vi "Main.vi"(11 "Module Admin":refnum<class "Delacor_lib_QMH_Module Admin.lvclass">) -> ()   [LabVIEW 2024, in "GUI.lvlib"]
doc: "This template is based off of the Queued Message Handler design pattern and the Queued Message Handler project template that ships with LabVIEW.\n\nThe main difference is that the queue is private to this module and communication between modules is performed via Broadcast and Request events.\n\nRequest events are wrapped in public API methods and are handled in the Event Handling Loop (EHL) of this VI. Any module can register for Broadcast events sent by this module. The EHL generates messages based on user interface actions.\n\nThe Message Handling Loop (MHL) processes messages generated by the EHL, or by other messages. The messages are string values, so new messages can be added easily to the Message Cases case structure in the MHL. Each message cluster can also provide an optional value for Message Data, which is a variant that can be converted to whatever message-specific data is required.\n_____\nBased on DQMH Dev Tools: Project Template 7.1.0.1503."
uses:
  GUI.lvlib
  <vilib>/Delacor/Delacor QMH/Libraries/Module Admin_class/Delacor_lib_QMH_Module Admin.lvclass
  DB/Controls/Login info.ctl
  DB/Controls/User level.ctl
  Controls/Main Buttons.ctl
  Controls/Settings.ctl
  <vilib>/vision/Instrument.llb/QR Code Description Options.ctl
  <vilib>/vision/Instrument.llb/Data Matrix Polarity.ctl
  <vilib>/vision/Instrument.llb/QR Code Model Type.ctl
  Controls/HW Status.ctl
  Module Data--cluster.ctl
  <vilib>/Delacor/Delacor QMH/Libraries/Message Queue_class/Delacor_lib_QMH_Message Queue.lvclass/Delacor_lib_QMH_Message Queue.ctl
  Stop Argument--cluster.ctl
  <vilib>/Delacor/Delacor QMH/Libraries/Module Admin_class/Delacor_lib_QMH_Module Admin.lvclass/Delacor_lib_QMH_Module Admin.ctl
  login Argument--cluster.ctl
  login_ Argument--cluster.ctl
  logout Argument--cluster.ctl
  Load settings Argument--cluster.ctl
  update serials array Argument--cluster.ctl
  update parent Argument--cluster.ctl
  update HW status indicator Argument--cluster.ctl
  Controls/HW Modules.ctl
  <vilib>/Utility/miscctls.llb/LVPointTypeDef.ctl
  GUI data ref.ctl
  <vilib>/Delacor/Delacor QMH/Libraries/Message Queue_class/Delacor_lib_QMH_Enqueue Message (Single).vi
  <vilib>/Delacor/Delacor QMH/Libraries/Module Admin_class/Delacor_lib_QMH_Get External Launch.vi
  <vilib>/Delacor/Delacor QMH/Libraries/Message Queue_class/Delacor_lib_QMH_Message Queue.lvclass
  DB/DB.lvlib
  Controller/Controller.lvlib
  PLC/PLC.lvlib
  Handheld Scanner/Handheld Scanner.lvlib
  Aggregation 1/Aggregation 1.lvlib
panel:
  in  "Close":bool
  in  "Back":bool
  out "Login info":T1
  in  "Tab Control":T3(tab)
  in  "Main buttons":T4
  out "Parent 2":string
  out "Parent 1":string
  in  "Start Tool":bool
  in  "Start Tool":bool
  out "Level 2 Serials":string[](array[string])
  out "Level 1 Serials":string[](array[string])
  out "Camera 2":T5(plugin-control)
  out "Camera 1":T5(plugin-control)
  out "Status":T6
  in  "Settings":T7
  in  "Cancel settings":bool
  in  "Save settings":bool
  out "Image":T5(plugin-control)
  in  "QR Search options":T8
  in  "QR Description Options":T9={"Matrix Size (cells)"=0, "Barcode Polarity"=-2, "Mirror Mode"=-2, "QR Model"=0} {"Mirror Mode" items=["Auto-detect"=-2, "Normal"=0, "Mirrored"=1]; "Matrix Size (cells)" items=["Auto-detect"=0, "11x11 - Version 1 (Micro QR Only)"=11, "13x13 - Version 2 (Micro QR Only)"=13, "15x15 - Version 3 (Micro QR Only)"=15, "17x17 - Version 4 (Micro QR Only)"=17, "21x21 - Version 1"=21, "25x25 - Version 2"=25, "29x29 - Version 3"=29, "33x33 - Version 4"=33, "37x37 - Version 5"=37, "41x41 - Version 6"=41, "45x45 - Version 7"=45, "49x49 - Version 8"=49, "53x53 - Version 9"=53, "57x57 - Version 10"=57, "61x61 - Version 11"=61, "65x65 - Version 12"=65, "69x69 - Version 13"=69, "73x73 - Version 14"=73, "77x77 - Version 15"=77, "81x81 - Version 16"=81, "85x85 - Version 17"=85, "89x89 - Version 18"=89, "93x93 - Version 19"=93, "97x97 - Version 20"=97, "101x101 - Version 21"=101, "105x105 - Version 22"=105, "109x109 - Version 23"=109, "113x113 - Version 24"=113, "117x117 - Version 25"=117, "121x121 - Version 26"=121, "125x125 - Version 27"=125, "129x129 - Version 28"=129, "133x133 - Version 29"=133, "137x137 - Version 30"=137, "141x141 - Version 31"=141, "145x145 - Version 32"=145, "149x149 - Version 33"=149, "153x153 - Version 34"=153, "157x157 - Version 35"=157, "161x161 - Version 36"=161, "165x165 - Version 37"=165, "169x169 -  Version 38"=169, "173x173 - Version 39"=173, "177x177 - Version 40"=177]; "QR Model" items=["Auto-detect", "Micro", "Model 1", "Model 2"]; "Barcode Polarity" items=["Auto-detect"=-2, "Black on White"=0, "White on Black"=1]}
  out "error out":errorcluster
  out "Status":string
  in  "Simulate MHL Error":bool
  in  "Simulate EHL Error":bool
  # "Other processes communicate with this Module via its Public API (wrappers for its Request Events).\n\nThis Module communicates with other processes via its Broadcast Events.\nAny process that wants to receive these messages can register for this module's Broadcast events."
  # "This template is for the DQMH framework. See the block diagram for more information on how to use this template."
  # "No User logged in\n        Or Database Not Connected\n\nPlease Login from Serialization System"
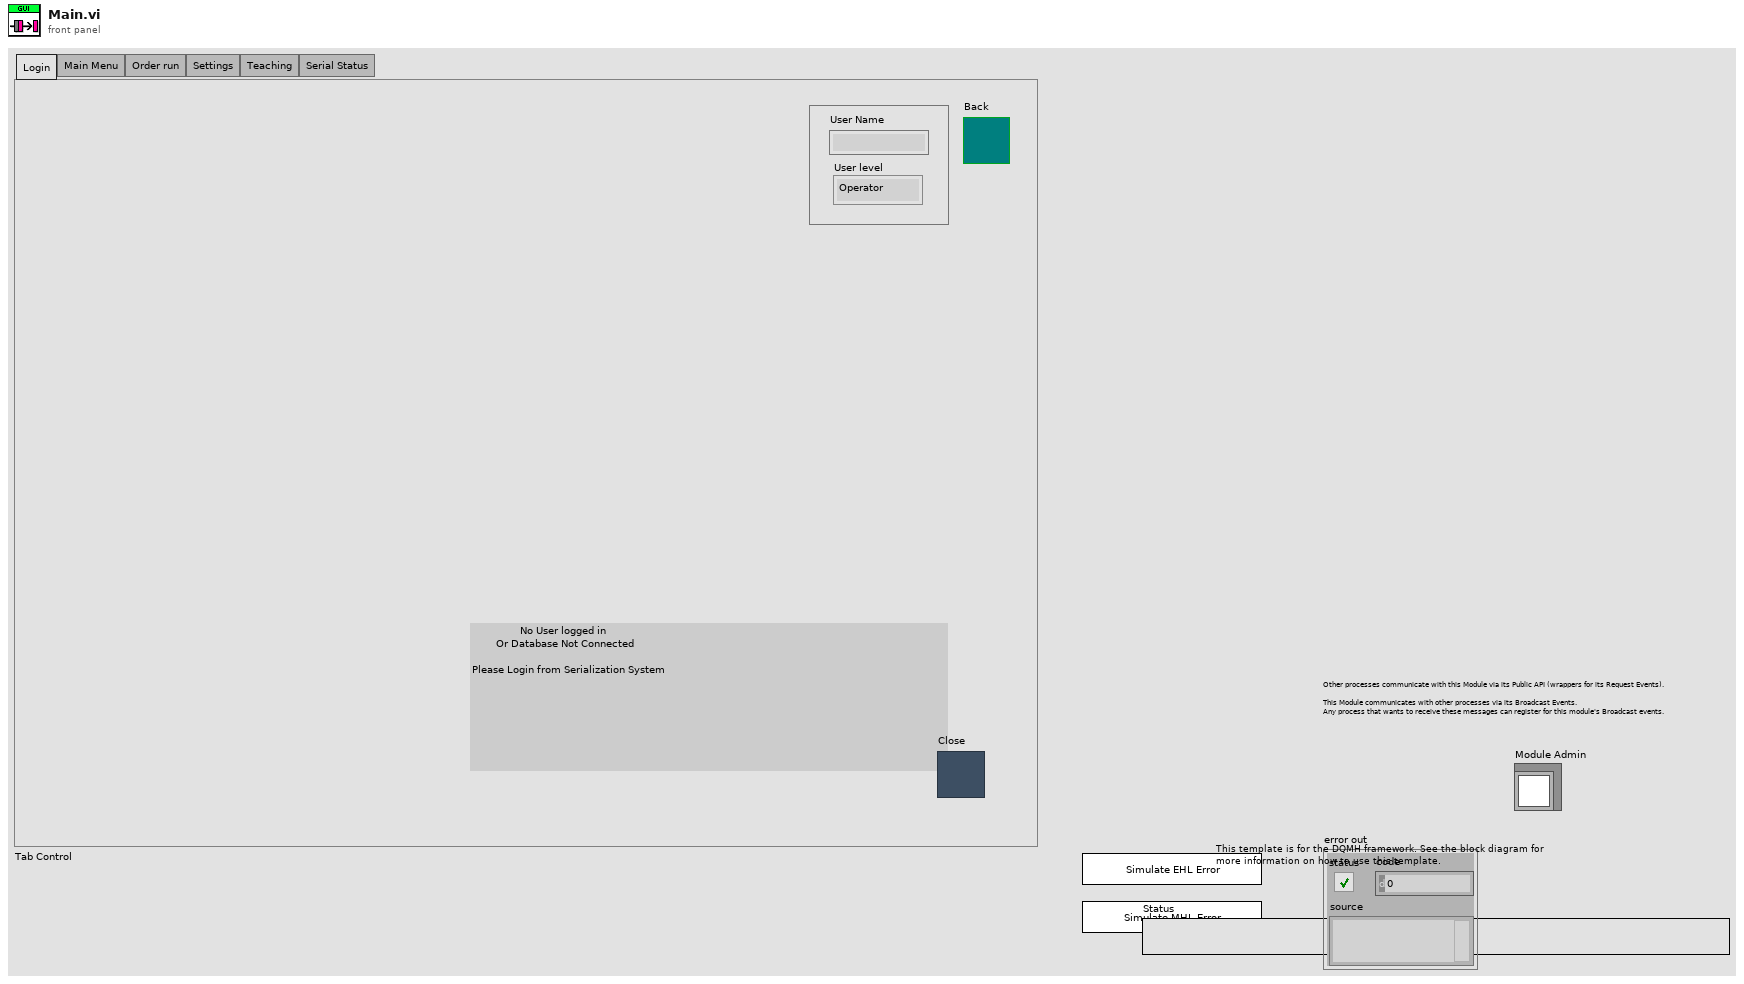
[diagram p1: front panel]
types:
  T1 = typedef "Login info.ctl" = cluster{"User Name":string, "User level":T2}
  T2 = typedef "User level.ctl" = enum16{"Operator", "Admin"}
  T3 = enum32{"Login", "Main Menu", "Order run", "Settings", "Teaching", "Serial Status"}
  T4 = typedef "Main Buttons.ctl" = cluster{"Start Button":bool, "Tools Button":bool, "Teaching Button":bool, "Serial Status Button":bool}
  T5 = typedef "IMAQ Image.ctl" = refnum<image>
  T6 = typedef "HW Status.ctl" = cluster{"Cam 1":bool, "Cam 2":bool, "Printer 1":bool, "Printer 2":bool, "PLC":bool, "Level 2 scanner":bool, "Handheld scanner":bool}
  T7 = typedef "Settings.ctl" = cluster{"Camera 1 IP":string, "Camera 2 IP":string, "Printer 1 IP":string, "Printer 2 IP":string, "Level 2 Scanner COM":refnum<visa-resource-name>, "PLC Port":dbl, "PLC IP":string, "Handheld Scanner COM":refnum<visa-resource-name>, "Printer2 Port":dbl, "Cam1 send port ":dbl, "Cam1 recv port":dbl, "Cam2 send port":dbl, "Cam recv port":dbl, "Printer1 Port":dbl}
  T8 = cluster{"Rotation Mode":enum32{"Unlimited", "0 Degrees", "90 Degrees", "180 Degrees", "270 Degrees"}, "Skip Location?":bool, "Edge Threshold":u32, "Demodulation Mode":i32, "Cell Sample Size":i32, "Cell Filter Mode":i32, "Skew Degrees Allowed":u32}
  T9 = typedef "QR Code Description Options.ctl" = cluster{"Matrix Size (cells)":i32, "Barcode Polarity":T10, "Mirror Mode":i32, "QR Model":T11}
  T10 = typedef "Data Matrix Polarity.ctl" = i32
  T11 = typedef "QR Code Model Type.ctl" = i32
  T12 = typedef "Controller.lvlib/Broadcast Events--cluster.ctl" = cluster{"Module Did Init":refnum<user-event>, "Status Updated":refnum<user-event>, "Error Reported":refnum<user-event>, "Module Did Stop":refnum<user-event>, "Update Module Execution Status":refnum<user-event>}
  T13 = typedef "DB.lvlib/Broadcast Events--cluster.ctl" = cluster{"Module Did Init":refnum<user-event>, "Status Updated":refnum<user-event>, "Error Reported":refnum<user-event>, "Module Did Stop":refnum<user-event>, "Update Module Execution Status":refnum<user-event>}
  T14 = typedef "PLC.lvlib/Broadcast Events--cluster.ctl" = cluster{"Module Did Init":refnum<user-event>, "Status Updated":refnum<user-event>, "Error Reported":refnum<user-event>, "Module Did Stop":refnum<user-event>, "Update Module Execution Status":refnum<user-event>}
  T15 = typedef "Aggregation 1.lvlib/Broadcast Events--cluster.ctl" = cluster{"Module Did Init":refnum<user-event>, "Status Updated":refnum<user-event>, "Error Reported":refnum<user-event>, "Module Did Stop":refnum<user-event>, "Update Module Execution Status":refnum<user-event>}
  T16 = typedef "Handheld Scanner.lvlib/Broadcast Events--cluster.ctl" = cluster{"Module Did Init":refnum<user-event>, "Status Updated":refnum<user-event>, "Error Reported":refnum<user-event>, "Module Did Stop":refnum<user-event>, "Update Module Execution Status":refnum<user-event>}
  T17 = typedef "GUI.lvlib/Request Events--cluster.ctl" = cluster{"Stop Module":refnum<user-event>, "Show Panel":refnum<user-event>, "Hide Panel":refnum<user-event>, "Get Module Execution Status":refnum<user-event>, "Show Diagram":refnum<user-event>, "login":refnum<user-event>, "login_":refnum<user-event>, "logout":refnum<user-event>, "Load settings":refnum<user-event>, "update serials array":refnum<user-event>, "update parent":refnum<user-event>, "update HW status indicator":refnum<user-event>}
  T18 = typedef "GUI.lvlib/Module Data--cluster.ctl" = cluster{"Status":string}
  T19 = enum32{"invalid lock state", "Not Locked", "Locked (No Password)", "Password-protected"}
  T20 = typedef "GUI.lvlib/Stop Argument--cluster.ctl" = cluster{"Origin":string, "Exit via Stop Module Req?":bool, "Wait for Module to stop?":bool}
  T21 = enum32{"Login", "Main Menu", "Order run", "Settings"}
  T22 = typedef "GUI.lvlib/login Argument--cluster.ctl" = cluster{"Login info":T1}
  T23 = typedef "GUI.lvlib/login_ Argument--cluster.ctl" = cluster{"Login info":T1}
  T24 = typedef "GUI.lvlib/logout Argument--cluster.ctl" = cluster{"Boolean":bool}
  T25 = typedef "GUI.lvlib/Load settings Argument--cluster.ctl" = cluster{"Settings":T7, "reconnect":bool}
  T26 = typedef "GUI.lvlib/update serials array Argument--cluster.ctl" = cluster{"serial array":string[], "level":dbl}
  T27 = typedef "GUI.lvlib/update parent Argument--cluster.ctl" = cluster{"Parent":string, "level":dbl}
  T28 = typedef "GUI.lvlib/update HW status indicator Argument--cluster.ctl" = cluster{"HW Module":T29, "Status":bool}
  T29 = typedef "HW Modules.ctl" = string
  T30 = typedef "LVPointTypeDef.ctl" = cluster{"Horizontal":i16, "Vertical":i16}
  T31 = enum32{"Invalid", "Standard", "Closed", "Hidden", "Minimized", "Maximized"}
  T32 = typedef "GUI data ref.ctl" = cluster{"Printer 1 IP":refnum<vi>, "Camera 2 IP":refnum<vi>, "Camera 1 IP":refnum<vi>, "Printer 2 IP":refnum<vi>}
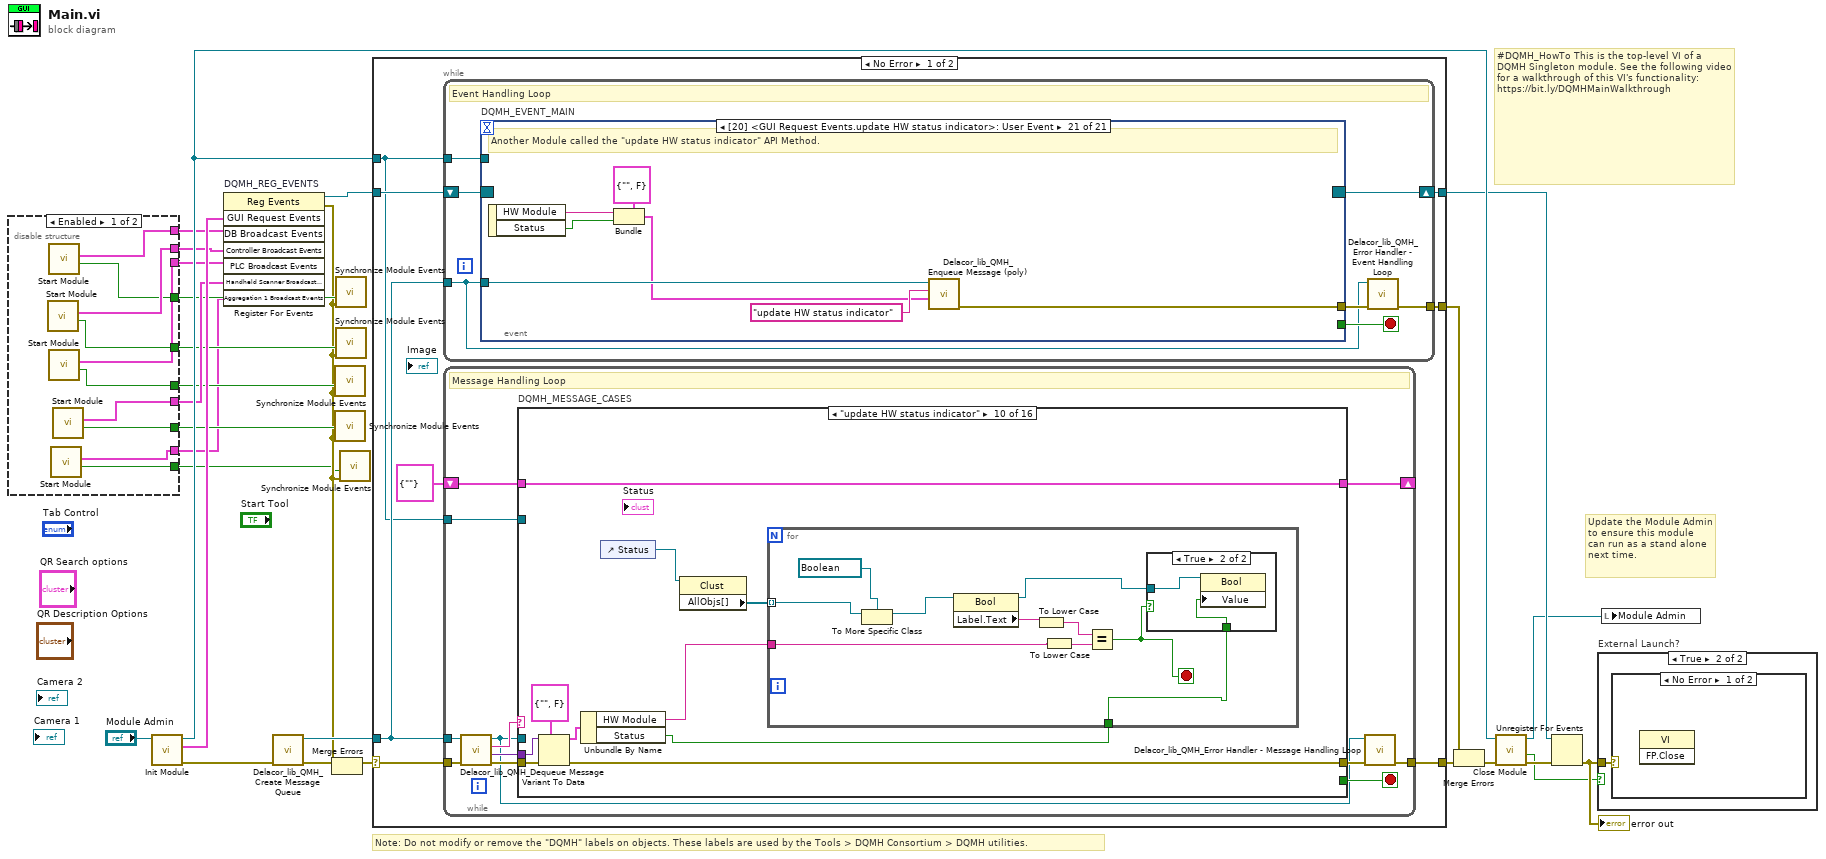
[diagram p0: block diagram]
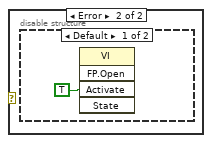
[diagram p4: hidden frame]
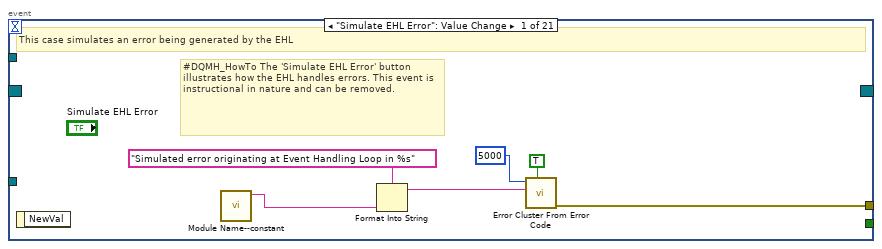
[diagram p6: hidden frame]
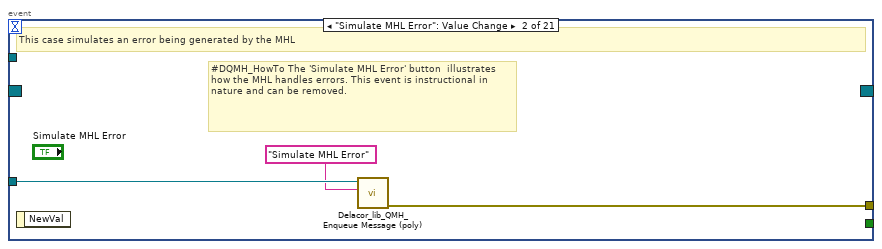
[diagram p7: hidden frame]
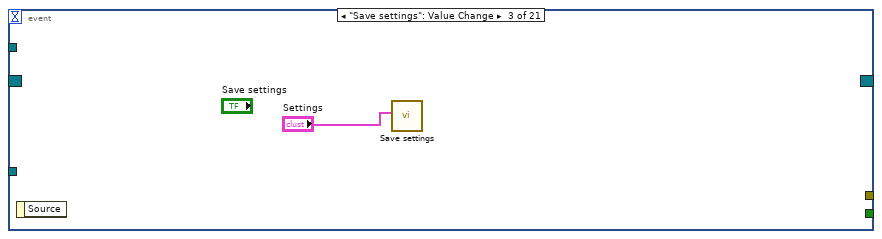
[diagram p8: hidden frame]
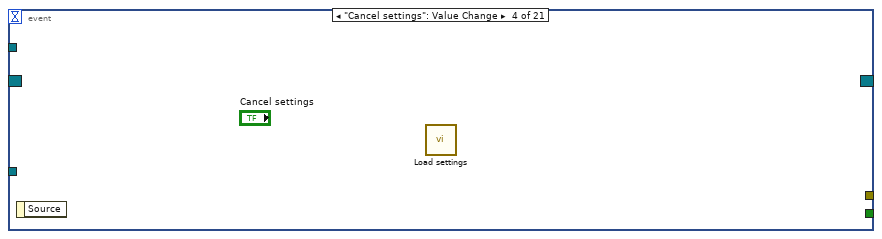
[diagram p9: hidden frame]
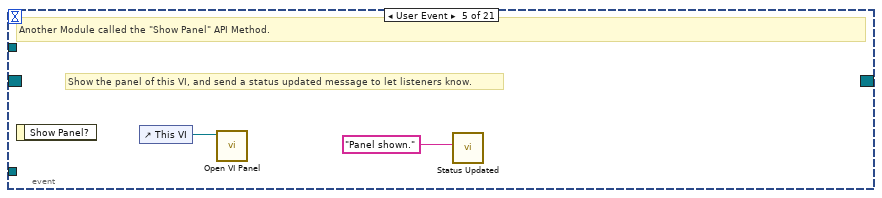
[diagram p10: hidden frame]
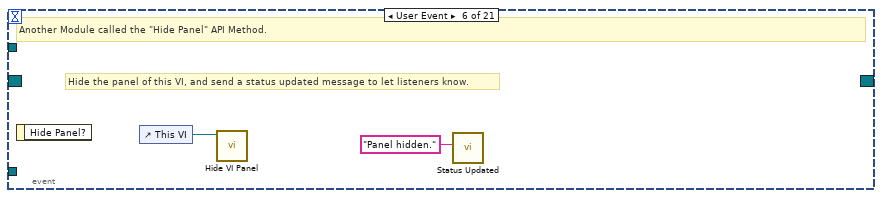
[diagram p11: hidden frame]
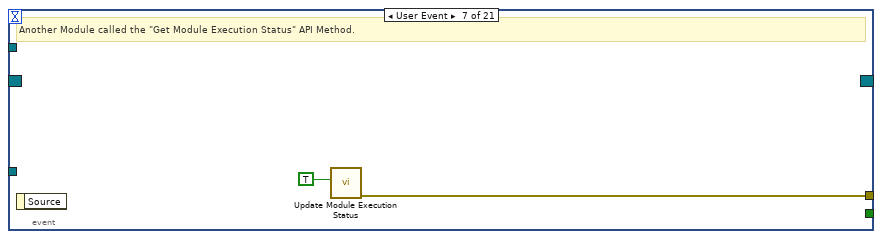
[diagram p12: hidden frame]
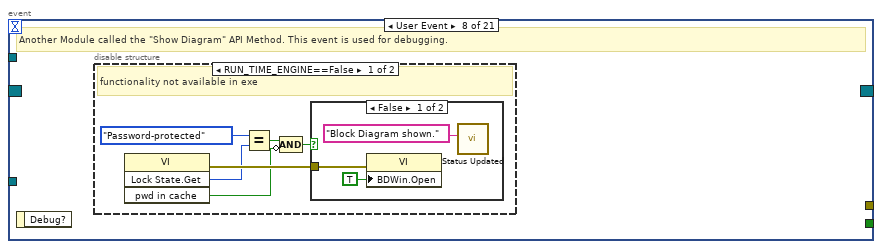
[diagram p13: hidden frame]
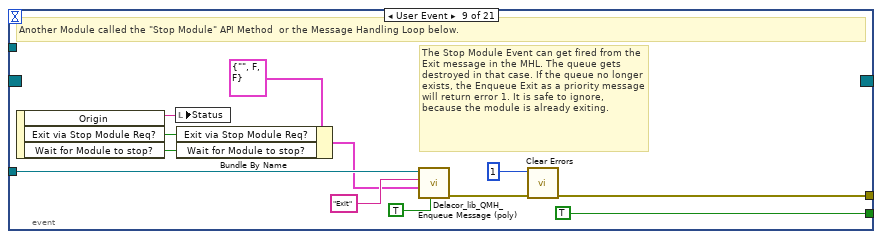
[diagram p16: hidden frame]
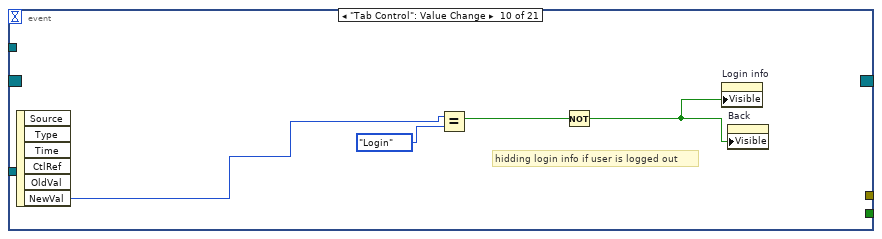
[diagram p17: hidden frame]
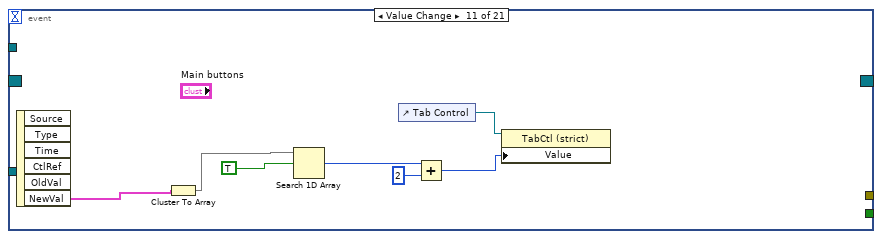
[diagram p18: hidden frame]
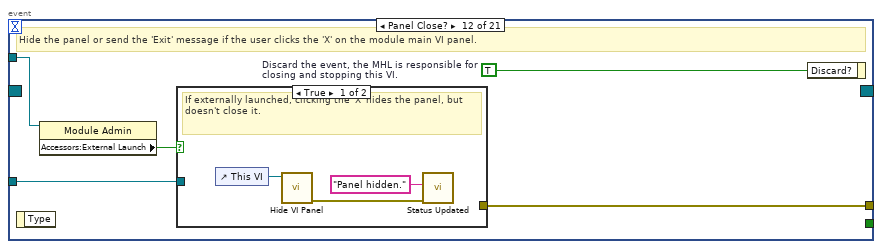
[diagram p19: hidden frame]
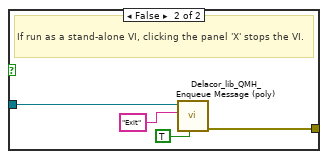
[diagram p20: hidden frame]
diagram:
  # "#DQMH_HowTo This is the top-level VI of a DQMH Singleton module. See the following video for a walkthrough of this VI's functionality: https://bit.ly/DQMHMainWalkthrough"
  # "Note: Do not modify or remove the \"DQMH\" labels on objects. These labels are used by the Tools > DQMH Consortium > DQMH utilities."
  # "Update the Module Admin to ensure this module can run as a stand alone next time."
  n1 = disable-structure shown="Enabled" {
    disable-tunnel: [w37 _] -> w11
    disable-tunnel: [w36 _] -> w10
    disable-tunnel: [w35 _] -> w9
    disable-tunnel: [w34 _] -> w8
    disable-tunnel: [w33 _] -> w7
    disable-tunnel: [w32 _] -> w6
    disable-tunnel: [w31 _] -> w5
    disable-tunnel: [w30 _] -> w4
    disable-tunnel: [w29 _] -> w2
    disable-tunnel: [w28 _] -> w1
    frame Enabled {
      n2 = call "Start Module.vi"() -> ("Wait for Event Sync?"=w32:bool, "Controller Broadcast Events"=w36:T12)  [unwired: 7 in, 3 out]
      n3 = call "Start Module.vi"() -> ("Wait for Event Sync?"=w33:bool, "DB Broadcast Events"=w37:T13)  [unwired: 7 in, 3 out]
      n4 = call "Start Module.vi"() -> ("Wait for Event Sync?"=w31:bool, "PLC Broadcast Events"=w35:T14)  [unwired: 7 in, 3 out]
      n5 = call "Start Module.vi"() -> ("Wait for Event Sync?"=w29:bool, "Aggregation 1 Broadcast Events"=w28:T15)  [unwired: 7 in, 3 out]
      n6 = call "Start Module.vi"() -> ("Wait for Event Sync?"=w30:bool, "Handheld Scanner Broadcast Events"=w34:T16)  [unwired: 7 in, 3 out]
    }
    frame Disabled {
    }
  }
  n7 = call "Init Module.vi"("Singleton Module Admin in"="Module Admin") -> ("error out"=w26:errorcluster, "GUI Request Events"=w16:T17, "Singleton Module Admin out"=w19:refnum<class "Delacor_lib_QMH_Module Admin.lvclass">)  [unwired: 8 in]
  n8 = register-events "DQMH_REG_EVENTS"(w16, w11, w10, w9, w8, w1) -> (reference out=w17:refnum<event-registration>, error out=w3:errorcluster)  [unwired: 2 in]
  n9 = call <vilib>:"Delacor_lib_QMH_Create Message Queue.vi"("error in"=w26) -> ("error out"=w21:errorcluster, "Message Queue"=w15:refnum<class "Delacor_lib_QMH_Message Queue.lvclass">)  [unwired: 9 in]
  n10 = Merge Errors(w21, w3) -> (w20:errorcluster)
  n11 = call "Synchronize Module Events.vi"("error in"=w3, "Wait for Event Sync?"=w5) -> ()  [unwired: 9 in, 1 out]
  n12 = call "Synchronize Module Events.vi"("error in"=w3, "Wait for Event Sync?"=w4) -> ()  [unwired: 9 in, 1 out]
  n13 = call "Synchronize Module Events.vi"("error in"=w3, "Wait for Event Sync?"=w7) -> ()  [unwired: 9 in, 1 out]
  n14 = call "Synchronize Module Events.vi"("error in"=w3, "Wait for Event Sync?"=w6) -> ()  [unwired: 9 in, 1 out]
  n15 = call "Synchronize Module Events.vi"("error in"=w3, "Wait for Event Sync?"=w2) -> ()  [unwired: 9 in, 1 out]
  n16 = case shown="No Error" w20 {
    selector: w20 -> [w43 w352]
    tunnel: [w45 w351] -> w27
    tunnel: [w42 w350] -> w18
    tunnel: w17 -> [w40 w350]
    tunnel: w15 -> [w39 w345]
    tunnel: [w44 _] -> w24
    tunnel: w19 -> [w38 w346]
    frame No Error {
      n17 = while {
        tunnel: w39 -> [w46]
        shift-right: [w49] -> w42
        shift-left: w40 -> [w50]
        tunnel: [w51] -> w44
        tunnel: w38 -> [w47]
        stop <- w48 stop-if-true
        # "Event Handling Loop"
        n18 = event "DQMH_EVENT_MAIN" shown="[20] <GUI Request Events.update HW status indicator>: User Event" {
          selector: w50 -> [_ _ _ _ _ _ _ _ _ _ _ _ _ _ _ _ _ _ _ _ _]
          dyn-events: [_ _ _ _ _ _ _ _ _ _ _ _ _ _ _ _ _ _ _ _ _] -> w49
          timeout: _ -> [_ _ _ _ _ _ _ _ _ _ _ _ _ _ _ _ _ _ _ _ _]
          tunnel: [_ _ _ _ _ _ _ _ TRUE ("Discard?") _ _ _ _ _ _ _ _ _ _ _ _] -> w48
          tunnel: w46 -> [_ w60 _ _ _ _ _ _ w85 _ _ w103 _ w118 w124 w130 _ w142 w149 w156 w163]
          tunnel: [w58 w61 _ _ _ _ w68 _ w88 _ _ w105 _ w113 w119 w125 _ w137 w143 w150 w157] -> w52
          tunnel: w47 -> [_ _ _ _ _ _ _ _ _ _ _ w102 _ _ _ _ _ _ _ _ _]
          event "Simulate EHL Error": Value Change {
            # "#DQMH_HowTo The 'Simulate EHL Error' button  illustrates how the EHL handles errors. This event is instructional in nature and can be removed."
            # "This case simulates an error being generated by the EHL"
            n19 = event-data() -> ()  [unwired: 1 in, 1 out]
            n20 = call "Module Name--constant.vi"() -> ("Module Name"=w55:string)  [unwired: 11 in]
            n21 = Format Into String(format string="Simulated error originating at Event Handling Loop in %s", w55) -> (resulting string=w56:string)  [unwired: 2 in, 1 out]
            n22 = call <vilib>:"Error Cluster From Error Code.vi"("show call chain? (False)"=TRUE, "error message (\"\")"=w56, "error code (0)"=5000) -> ("error out"=w58:errorcluster)  [unwired: 6 in]
          }
          event "Simulate MHL Error": Value Change {
            # "#DQMH_HowTo The 'Simulate MHL Error' button  illustrates how the MHL handles errors. This event is instructional in nature and can be removed."
            # "This case simulates an error being generated by the MHL"
            n23 = event-data() -> ()  [unwired: 1 in, 1 out]
            n24 = call-poly <vilib>:"Delacor_lib_QMH_Enqueue Message (poly).vi"("Message"="Simulate MHL Error", "Message Queue in"=w60) -> ("error out"=w61:errorcluster)  [unwired: 8 in, 1 out]
          }
          event "Save settings": Value Change {
            n25 = event-data() -> ()  [unwired: 1 in, 1 out]
            n26 = call "Save settings.vi"("Settings"="Settings") -> ()  [unwired: 10 in, 1 out]
          }
          event "Cancel settings": Value Change {
            n27 = event-data() -> ()  [unwired: 1 in, 1 out]
            n28 = call "Load settings.vi"() -> ()  [unwired: 11 in, 1 out]
          }
          event User Event {
            # "Show the panel of this VI, and send a status updated message to let listeners know."
            # "Another Module called the \"Show Panel\" API Method."
            n29 = event-data() -> ()  [unwired: 1 in, 1 out]
            n30 = control-ref of="This VI"() -> (w64:refnum<vi>)
            n31 = call "Open VI Panel.vi"("VI"=w64) -> ()  [unwired: 10 in, 1 out]
            n32 = call "Status Updated.vi"("Status"="Panel shown." ("format string")) -> ()  [unwired: 10 in, 1 out]
          }
          event User Event {
            # "Hide the panel of this VI, and send a status updated message to let listeners know."
            # "Another Module called the \"Hide Panel\" API Method."
            n33 = event-data() -> ()  [unwired: 1 in, 1 out]
            n34 = control-ref of="This VI"() -> (w66:refnum<vi>)
            n35 = call "Hide VI Panel.vi"("VI"=w66) -> ()  [unwired: 10 in, 1 out]
            n36 = call "Status Updated.vi"("Status"="Panel hidden." ("format string")) -> ()  [unwired: 10 in, 1 out]
          }
          event User Event {
            # "Another Module called the \"Get Module Execution Status\" API Method."
            n37 = event-data() -> ()  [unwired: 1 in, 1 out]
            n38 = call "Update Module Execution Status.vi"("Running?"=TRUE) -> ("error out"=w68:errorcluster)  [unwired: 10 in]
          }
          event User Event {
            # "Another Module called the \"Show Diagram\" API Method. This event is used for debugging."
            n39 = event-data() -> ()  [unwired: 1 in, 1 out]
            n40 = disable-structure shown="RUN_TIME_ENGINE==False" {
              frame condition #0 (active) {
                # "functionality not available in exe"
                n41 = invoke on="Invoke Node" class="VI" method="Lock State.Get"() -> (error out=w74:errorcluster, "Get Lock State"=w73:T19, "pwd in cache"=w70:bool)  [unwired: 4 in, 1 out]
                n42 = Equal?(x=T19."Password-protected", y=w73) -> (x = y?=w71:bool)
                n43 = Compound Arithmetic op=AND(w71, invert w70) -> (w69:bool)
                n44 = case shown="False" w69 {
                  tunnel: w74 -> [w77 _]
                  frame False {
                    n45 = property on="Property Node" class="VI"(error in=w77, "BDWin.Open"=TRUE ("Block Diagram Window:Open")) -> ()  [unwired: 1 in, 2 out]
                    n46 = call "Status Updated.vi"("Status"="Block Diagram shown." ("format string")) -> ()  [unwired: 10 in, 1 out]
                  }
                  frame True {
                    # "Password-protected VI, and the password is not in the cache. Do not show the diagram."
                  }
                }
              }
              frame condition #1 {
              }
            }
          }
          event User Event {
            # "The Stop Module Event can get fired from the Exit message in the MHL. The queue gets destroyed in that case. If the queue no longer exists, the Enqueue Exit as a priority message will return error 1. It is safe to ignore, because the module is already exiting."
            # "Another Module called the \"Stop Module\" API Method  or the Message Handling Loop below."
            n47 = event-data() -> ("Origin"=w84:string, "Exit via Stop Module Req?"=w80:bool, "Wait for Module to stop?"=w79:bool)  [unwired: 1 in]
            n48 = local write "Status"(w84) -> ()
            n49 = Bundle By Name(cluster=T20 {"Origin"="", "Exit via Stop Module Req?"=FALSE, "Wait for Module to stop?"=FALSE} ("Stop Argument"), "Exit via Stop Module Req?"=w80, "Wait for Module to stop?"=w79) -> (w78:T20)
            n50 = call-poly <vilib>:"Delacor_lib_QMH_Enqueue Message (poly).vi"("Priority Message? (F)"=TRUE, "Message Data"=w78, "Message"="Exit", "Message Queue in"=w85) -> ("error out"=w89:errorcluster)  [unwired: 6 in, 1 out]
            n51 = call <vilib>:"Clear Errors.vi"("error in (no error)"=w89, "specific error code to clear (0: all)"=1) -> ("error out"=w88:errorcluster)  [unwired: 4 in, 1 out]
          }
          event "Tab Control": Value Change {
            # "hidding login info if user is logged out"
            n52 = event-data() -> ("NewVal"=w93:T3)  [unwired: 1 in, 5 out]
            n53 = Equal?(x=w93, y=T21."Login") -> (x = y?=w91:bool)
            n54 = Not(x=w91) -> (.not. x?=w90:bool)
            n55 = property on="Login info" class="Clust (strict)"("Visible"=w90) -> ()  [unwired: 2 in, 2 out]
            n56 = property on="Back" class="Bool"("Visible"=w90) -> ()  [unwired: 2 in, 2 out]
          }
          event Value Change {
            n57 = event-data() -> ("NewVal"=w100:T4)  [unwired: 1 in, 5 out]
            n58 = Cluster To Array(cluster=w100) -> (array=w99:bool[])
            n59 = Search 1D Array(1D array=w99, element=TRUE) -> (index of element=w97:i32)  [unwired: 1 in]
            n60 = control-ref of="Tab Control"() -> (w94:refnum<vi>)
            n61 = Add(x=w97, y=2) -> (x+y=w95:i32)
            n62 = property class="TabCtl (strict)"(reference=w94, "Value"=w95) -> ()  [unwired: 1 in, 2 out]
          }
          event Panel Close? {
            w104 = TRUE  # Discard the event, the MHL is responsible for closing and stopping this VI.
            # "Hide the panel or send the 'Exit' message if the user clicks the 'X' on the module main VI panel."
            n63 = event-data() -> ()  [unwired: 1 in, 1 out]
            n64 = property on="Property Node" class="Module Admin"(reference=w102) -> ("Accessors:External Launch"=w101:bool)  [unwired: 1 in, 2 out]
            n65 = case shown="True" w101 {
              tunnel: w103 -> [_ w111]
              tunnel: [_ w112] -> w105
              frame True {
                # "If externally launched, clicking the 'X' hides the panel, but doesn't close it."
                n66 = control-ref of="This VI"() -> (w108:refnum<vi>)
                n67 = call "Hide VI Panel.vi"("VI"=w108) -> ("error out"=w106:errorcluster)  [unwired: 10 in]
                n68 = call "Status Updated.vi"("error in"=w106, "Status"="Panel hidden." ("format string")) -> ()  [unwired: 9 in, 1 out]
              }
              frame False {
                # "If run as a stand-alone VI, clicking the panel 'X' stops the VI."
                n69 = call-poly <vilib>:"Delacor_lib_QMH_Enqueue Message (poly).vi"("Priority Message? (F)"=TRUE, "Message"="Exit", "Message Queue in"=w111) -> ("error out"=w112:errorcluster)  [unwired: 7 in, 1 out]
              }
            }
            n70 = event-data ("Event Filter Node")("Discard?"=w104) -> ()  [unwired: 1 in, 1 out]
          }
          event "Close": Value Change {
            n71 = event-data() -> ()  [unwired: 1 in, 1 out]
            n72 = call "Stop Module.vi"() -> ()  [unwired: 11 in, 1 out]
          }
          event User Event {
            # "Another Module called the \"login\" API Method."
            n73 = event-data() -> ("Login info"=w114:T1)  [unwired: 1 in]
            n74 = Bundle(cluster=T22 {"Login info"={"User Name"="", "User level"=enum."Operator"}} ("login Argument"), "Login info"=w114) -> (w115:T22)
            n75 = call-poly <vilib>:"Delacor_lib_QMH_Enqueue Message (poly).vi"("Message Data"=w115, "Message"="login", "Message Queue in"=w118) -> ("error out"=w113:errorcluster)  [unwired: 7 in, 1 out]
          }
          event User Event {
            # "Another Module called the \"login_\" API Method."
            n76 = event-data() -> ("Login info"=w120:T1)  [unwired: 1 in]
            n77 = Bundle(cluster=T23 {"Login info"={"User Name"="", "User level"=enum."Operator"}} ("login_ Argument"), "Login info"=w120) -> (w121:T23)
            n78 = call-poly <vilib>:"Delacor_lib_QMH_Enqueue Message (poly).vi"("Message Data"=w121, "Message"="login_", "Message Queue in"=w124) -> ("error out"=w119:errorcluster)  [unwired: 7 in, 1 out]
          }
          event User Event {
            # "Another Module called the \"logout\" API Method."
            n79 = event-data() -> ("Boolean"=w126:bool)  [unwired: 1 in]
            n80 = Bundle(cluster=T24 {"Boolean"=FALSE} ("logout Argument"), "Boolean"=w126) -> (w127:T24)
            n81 = call-poly <vilib>:"Delacor_lib_QMH_Enqueue Message (poly).vi"("Message Data"=w127, "Message"="logout", "Message Queue in"=w130) -> ("error out"=w125:errorcluster)  [unwired: 7 in, 1 out]
          }
          event "Back": Value Change {
            n82 = event-data() -> ()  [unwired: 1 in, 6 out]
            n83 = control-ref of="Tab Control"() -> (w133:refnum<vi>)
            n84 = property class="TabCtl (strict)"(reference=w133) -> (reference out=w131:refnum<vi>, "Value"=w132:T3)  [unwired: 1 in, 1 out]
            n85 = case shown="Default" w132 {
              tunnel: w131 -> [w135 _]
              frame Default {
                n86 = property class="TabCtl (strict)"(reference=w135, "Value"=T3."Main Menu") -> ()  [unwired: 1 in, 2 out]
              }
              frame "Login", "Main Menu" {
              }
            }
          }
          event User Event {
            # "Another Module called the \"Load settings\" API Method."
            n87 = event-data() -> ("Settings"=w138:T7, "reconnect"=w136:bool)  [unwired: 1 in]
            n88 = Bundle(cluster=T25 {"Settings"={"Camera 1 IP"="", "Camera 2 IP"="", "Printer 1 IP"="", "Printer 2 IP"="", "Level 2 Scanner COM"="", "PLC Port"=0.0, "PLC IP"="", "Handheld Scanner COM"="", "Printer2 Port"=0.0, "Cam1 send port "=0.0, "Cam1 recv port"=0.0, "Cam2 send port"=0.0, "Cam recv port"=0.0, "Printer1 Port"=0.0}, "reconnect"=FALSE} ("Load settings Argument"), "Settings"=w138, "reconnect"=w136) -> (w139:T25)
            n89 = call-poly <vilib>:"Delacor_lib_QMH_Enqueue Message (poly).vi"("Message Data"=w139, "Message"="Load settings", "Message Queue in"=w142) -> ("error out"=w137:errorcluster)  [unwired: 7 in, 1 out]
          }
          event User Event {
            # "Another Module called the \"update serials array\" API Method."
            n90 = event-data() -> ("serial array"=w145:string[], "level"=w144:dbl)  [unwired: 1 in]
            n91 = Bundle(cluster=T26 {"serial array"=[], "level"=0.0} ("update serials array Argument"), "serial array"=w145, "level"=w144) -> (w146:T26)
            n92 = call-poly <vilib>:"Delacor_lib_QMH_Enqueue Message (poly).vi"("Message Data"=w146, "Message"="update serials array", "Message Queue in"=w149) -> ("error out"=w143:errorcluster)  [unwired: 7 in, 1 out]
          }
          event User Event {
            # "Another Module called the \"update parent\" API Method."
            n93 = event-data() -> ("Parent"=w152:string, "level"=w151:dbl)  [unwired: 1 in]
            n94 = Bundle(cluster=T27 {"Parent"="", "level"=0.0} ("update parent Argument"), "Parent"=w152, "level"=w151) -> (w153:T27)
            n95 = call-poly <vilib>:"Delacor_lib_QMH_Enqueue Message (poly).vi"("Message Data"=w153, "Message"="update parent", "Message Queue in"=w156) -> ("error out"=w150:errorcluster)  [unwired: 7 in, 1 out]
          }
          event User Event {
            # "Another Module called the \"update HW status indicator\" API Method."
            n96 = event-data() -> ("HW Module"=w159:T29, "Status"=w158:bool)  [unwired: 1 in]
            n97 = Bundle(cluster=T28 {"HW Module"="", "Status"=FALSE} ("update HW status indicator Argument"), "HW Module"=w159, "Status"=w158) -> (w160:T28)
            n98 = call-poly <vilib>:"Delacor_lib_QMH_Enqueue Message (poly).vi"("Message Data"=w160, "Message"="update HW status indicator", "Message Queue in"=w163) -> ("error out"=w157:errorcluster)  [unwired: 7 in, 1 out]
          }
        }
        n99 = call-dynamic "Delacor_lib_QMH_Error Handler - Event Handling Loop.vi"("error in"=w52, "Message Queue in"=w46) -> ("dup error in"=w51:errorcluster)  [unwired: 8 in, 1 out]
      }
      n100 = while {
        tunnel: w39 -> [w164]
        shift-right: [w172] -> _
        shift-left: T18 {"Status"=""} ("Data Cluster") -> [w173]
        tunnel: w43 -> [w175]
        tunnel: [w167] -> w45
        tunnel: w38 -> [w168]
        stop <- w171 stop-if-true
        # "Message Handling Loop"
        n101 = call-dynamic "Delacor_lib_QMH_Dequeue Message.vi"("error in"=w175, "Message Queue in"=w164) -> ("error out"=w174:errorcluster, "Message Data"=w169:variant, "Message"=w170:string, "Message Queue out"=w165:refnum<class "Delacor_lib_QMH_Message Queue.lvclass">)  [unwired: 6 in]
        n102 = case "DQMH_MESSAGE_CASES" shown="\"update HW status indicator\"" w170 {
          selector: w170 -> [_ _ _ _ _ _ _ _ _ _ _ _ _ _ _ w340]
          tunnel: w165 -> [w177 _ _ _ _ _ _ _ _ _ _ _ _ w306 w328 _]
          tunnel: w174 -> [w197 w204 w214 w216 w226 w237 w245 w254 w264 w276 w291 w293 w302 w313 w334 w343]
          tunnel: [w195 w204 w214 w216 w224 w235 w243 w252 w262 w274 w290 w293 w301 w309 w329 w344] -> w166
          tunnel: w173 -> [w186 w203 w213 w215 w225 w236 w244 w253 w263 w275 w289 w292 w299 w308 w327 w341]
          tunnel: [w185 w203 w213 w215 w225 w236 w244 w253 w263 w275 w289 w292 w299 w308 w327 w341] -> w172
          tunnel: [_ _ _ _ _ _ _ _ _ _ _ _ _ _ w326 _] -> w171
          tunnel: w169 -> [_ _ _ _ w223 w234 w242 w251 w261 w273 _ _ _ w307 w325 _]
          tunnel: w168 -> [w187 _ _ _ _ _ _ _ _ _ _ _ _ w305 w320 _]
          frame "Initialize" {
            w181 = "Initial Message" ("Initial Message")
            # "#DQMH_CodeNeeded - Initialize the appearance of the front panel."
            # "#DQMH_CodeNeeded - Initialize your state data here."
            # "Initialize - Any operation that needs to be done before the module can receive messages. Synchronize Caller Events.vi will inform Start Module.vi that the module has launched and is ready to receive messages. Module Did Init.vi will broadcast that the module initialized."
            n103 = call "Synchronize Caller Events.vi"("error in"=w197, "Singleton Module Admin in"=w187) -> ("error out"=w196:errorcluster, "Singleton Module Admin out"=w182:refnum<class "Delacor_lib_QMH_Module Admin.lvclass">)  [unwired: 8 in]
            n104 = property on="Property Node" class="Module Admin"(reference=w182) -> ("Accessors:External Launch"=w191:bool)  [unwired: 1 in, 2 out]
            n105 = Select(t=T31."Hidden" ("State"), s=w191, f=T31."Standard" ("State")) -> (s? t:f=w188:T31)
            n106 = call "Module Name--constant.vi"() -> ("Module Name"=w194:string)  [unwired: 11 in]
            n107 = property on="Property Node" class="VI"("Front Panel.Title"=w194) -> (reference out=w193:refnum<vi>, error out=w199:errorcluster)  [unwired: 2 in]
            n108 = invoke on="Invoke Node" class="VI" method="FP.Open"(reference=w193, error in=w199, "State"=w188) -> (reference out=w192:refnum<vi>, error out=w198:errorcluster)  [unwired: 2 in, 3 out]
            n109 = Bundle By Name(cluster=w186, "Status"=w181) -> (w185:T18)
            n110 = invoke on="Invoke Node" class="VI" method="FP.Center"(reference=w192, error in=w198) -> ()  [unwired: 1 in, 3 out]
            n111 = property on="Pane" class="Pane"("Origin"=T30 {"Horizontal"=0, "Vertical"=0}) -> ()  [unwired: 2 in, 2 out]
            n112 = call-poly <vilib>:"Delacor_lib_QMH_Enqueue Message (poly).vi"("Message"="GUI init", "Message Queue in"=w177) -> ("Message Queue out"=w176:refnum<class "Delacor_lib_QMH_Message Queue.lvclass">)  [unwired: 8 in, 1 out]
            n113 = call "Module Name--constant.vi"() -> ("Module Name"=w183:string)  [unwired: 11 in]
            n114 = call-poly <vilib>:"Delacor_lib_QMH_Enqueue Message (poly).vi"("Message"="update ref", "Message Queue in"=w176) -> ()  [unwired: 8 in, 2 out]
            n115 = call "Module Did Init.vi"("error in"=w196, "Initialized?"=TRUE, "Origin"=w183) -> ("error out"=w195:errorcluster)  [unwired: 8 in]
            "Status" <- w181
          }
          frame "GUI init" {
            w202 = FALSE
            # "initializing buttons"
            n116 = disable-structure shown="RUN_TIME_ENGINE==True" {
              disable-tunnel: [TRUE FALSE] -> w201
              frame condition #0 (active) {
              }
              frame condition #1 {
              }
            }
            n117 = property on="Tab Control" class="TabCtl (strict)"("Tabs Visible?"=w201) -> ()  [unwired: 2 in, 2 out]
            n118 = property on="Login info" class="Clust (strict)"("Visible"=w202) -> ()  [unwired: 2 in, 2 out]
            n119 = property on="Back" class="Bool"("Visible"=w202) -> ()  [unwired: 2 in, 2 out]
            n120 = property on="Tab Control" class="TabCtl (strict)"("Value"=T3."Login" ("Tab Control")) -> ()  [unwired: 2 in, 2 out]
          }
          frame "update ref" {
            n121 = control-ref of="Printer 1 IP"() -> (w210:refnum<vi>)
            n122 = control-ref of="Camera 2 IP"() -> (w209:refnum<vi>)
            n123 = control-ref of="Camera 1 IP"() -> (w208:refnum<vi>)
            n124 = control-ref of="Printer 2 IP"() -> (w207:refnum<vi>)
            n125 = Bundle By Name(cluster=T32 {"Printer 1 IP"=refnum, "Camera 2 IP"=refnum, "Camera 1 IP"=refnum, "Printer 2 IP"=refnum} ("Cluster"), "Printer 1 IP"=w210, "Camera 2 IP"=w209, "Camera 1 IP"=w208, "Printer 2 IP"=w207) -> (w212:T32)
            n126 = call "Update References.vi"("Cluster"=w212) -> ()  [unwired: 10 in, 1 out]
          }
          frame "---Module Specific---" {
            # "Separator -- The following cases handle messages specific to this Module."
          }
          frame "login_" {
            # "this event is generated by DB module when user is logged in"
            n127 = Variant To Data(error in=w226, type=T22 {"Login info"={"User Name"="", "User level"=enum."Operator"}} ("login Argument"), Variant=w223) -> (data=w221:T22, error out=w224:errorcluster)
            n128 = Unbundle By Name(w221) -> ("Login info"=w217:T1)
            n129 = control-ref of="Tab Control"() -> (w220:refnum<vi>)
            n130 = property class="TabCtl (strict)"(reference=w220) -> (reference out=w218:refnum<vi>, "Value"=w219:T3)  [unwired: 1 in, 1 out]
            n131 = case shown="\"Login\"" w219 {
              tunnel: w218 -> [w229 _]
              tunnel: w217 -> [w227 _]
              frame "Login" {
                n132 = property class="TabCtl (strict)"(reference=w229, "Val(Sgnl)"=T21."Main Menu" ("Value")) -> ()  [unwired: 1 in, 2 out]
                "Login info" <- w227
              }
              frame "Main Menu", Default {
              }
            }
          }
          frame "logout" {
            n133 = Variant To Data(error in=w237, type=T24 {"Boolean"=FALSE} ("logout Argument"), Variant=w234) -> (data=w232:T24, error out=w235:errorcluster)
            n134 = Unbundle By Name(w232) -> ()  [unwired: 1 out]
            n135 = control-ref of="Tab Control"() -> (w231:refnum<vi>)
            n136 = property class="TabCtl (strict)"(reference=w231, "Val(Sgnl)"=T3."Login" ("Value (Signaling)")) -> ()  [unwired: 1 in, 2 out]
          }
          frame "Load settings" {
            n137 = Variant To Data(error in=w245, type=T25 {"Settings"={"Camera 1 IP"="", "Camera 2 IP"="", "Printer 1 IP"="", "Printer 2 IP"="", "Level 2 Scanner COM"="", "PLC Port"=0.0, "PLC IP"="", "Handheld Scanner COM"="", "Printer2 Port"=0.0, "Cam1 send port "=0.0, "Cam1 recv port"=0.0, "Cam2 send port"=0.0, "Cam recv port"=0.0, "Printer1 Port"=0.0}, "reconnect"=FALSE} ("Load settings Argument"), Variant=w242) -> (data=w240:T25, error out=w243:errorcluster)
            n138 = Unbundle By Name(w240) -> ("reconnect"=w239:bool, "Settings"=w238:T7)
            n139 = property on="Settings" class="Clust (strict)"("Value"=w238) -> ()  [unwired: 2 in, 2 out]
            n140 = case shown="True" w239 {
              tunnel: w238 -> [_ w246]
              frame False {
              }
              frame True {
                # "reconnect all modules"
                n141 = call "connect all modules.vi"("Settings"=w246) -> ()  [unwired: 10 in, 1 out]
              }
            }
          }
          frame "update serials array" {
            n142 = Variant To Data(error in=w254, type=T26 {"serial array"=[], "level"=0.0} ("update serials array Argument"), Variant=w251) -> (data=w249:T26, error out=w252:errorcluster)
            n143 = Unbundle By Name(w249) -> ("serial array"=w247:string[], "level"=w248:dbl)
            n144 = case shown="2" w248 {
              tunnel: w247 -> [_ w255 w256]
              frame 0, Default {
              }
              frame 1 {
                "Level 1 Serials" <- w255
              }
              frame 2 {
                "Level 2 Serials" <- w256
              }
            }
          }
          frame "update parent" {
            n145 = Variant To Data(error in=w264, type=T27 {"Parent"="", "level"=0.0} ("update parent Argument"), Variant=w261) -> (data=w259:T27, error out=w262:errorcluster)
            n146 = Unbundle By Name(w259) -> ("Parent"=w258:string, "level"=w257:dbl)
            n147 = case shown="1" w257 {
              tunnel: w258 -> [_ w265 w266]
              frame 0, Default {
              }
              frame 1 {
                "Parent 1" <- w265
              }
              frame 2 {
                "Parent 2" <- w266
              }
            }
          }
          frame "update HW status indicator" {
            n148 = Variant To Data(error in=w276, type=T28 {"HW Module"="", "Status"=FALSE} ("update HW status indicator Argument"), Variant=w273) -> (data=w271:T28, error out=w274:errorcluster)
            n149 = Unbundle By Name(w271) -> ("HW Module"=w268:T29, "Status"=w267:bool)
            n150 = control-ref of="Status"() -> (w270:refnum<vi>)
            n151 = property class="Clust"(reference=w270) -> ("AllObjs[]"=w269:refnum<vi>[])  [unwired: 1 in, 2 out]
            n152 = for {
              tunnel: w269 -> [w286] mode=indexing
              tunnel: w268 -> [w282]
              tunnel: w267 -> [w278]
              stop <- w277 stop-if-true
              n153 = To More Specific Class(target class=refnum<vi> refnum ("Cam 2"), reference=w286) -> (specific class reference=w284:refnum<vi>)  [unwired: 1 in, 1 out]
              n154 = property class="Bool"(reference=w284) -> (reference out=w279:refnum<vi>, "Label.Text"=w283:string)  [unwired: 1 in, 1 out]
              n155 = To Lower Case(string=w283) -> (all lower case string=w281:string)
              n156 = To Lower Case(string=w282) -> (all lower case string=w280:T29)
              n157 = Equal?(x=w281, y=w280) -> (x = y?=w277:bool)
              n158 = case shown="True" w277 {
                tunnel: w279 -> [_ w288]
                tunnel: w278 -> [_ w287]
                frame False {
                }
                frame True {
                  n159 = property class="Bool"(reference=w288, "Value"=w287) -> ()  [unwired: 1 in, 2 out]
                }
              }
            }
          }
          frame "---Copy This Frame---" {
            # "Duplicate this frame when creating new messages.  Change this comment in the duplicated frame to describe this message."
            n160 = Merge Errors(w291) -> (w290:errorcluster)
          }
          frame "---Exit and Error Handling---" {
            # "Separator - The following cases handle errors and exit messages."
          }
          frame "Simulate MHL Error" {
            # "#DQMH_HowTo The 'Simulate MHL Error' button  illustrates how the MHL handles errors. This event is instructional in nature and can be removed."
            # "Simulate an error occurring at the MHL"
            n161 = call "Module Name--constant.vi"() -> ("Module Name"=w295:string)  [unwired: 11 in]
            n162 = Format Into String(format string="Simulated error originating at Message Handling Loop in %s", w295) -> (resulting string=w296:string)  [unwired: 2 in, 1 out]
            n163 = call <vilib>:"Error Cluster From Error Code.vi"("show call chain? (False)"=TRUE, "error message (\"\")"=w296, "error code (0)"=5001) -> ("error out"=w300:errorcluster)  [unwired: 6 in]
            n164 = Merge Errors(w302, w300) -> (w301:errorcluster)
          }
          frame "Error" {
            # "#DQMH_CodeRecommended - If the module is running in standalone mode (External Launch = FALSE), this code will pop up an error dialog and call the 'Exit' message if an error occurs. Add more fine-grained error management here."
            # "Error - Check the error message data and respond accordingly. This message is sent by the \"Error Handler\" VIs at the end of each loop in this application."
            n165 = property on="Property Node" class="Module Admin"(reference=w305) -> ("Accessors:External Launch"=w304:bool)  [unwired: 1 in, 2 out]
            n166 = Variant To Data(error in=w313, type=errorcluster {"status"=FALSE, "code"=0, "source"=""} ("error constant"), Variant=w307) -> (data=w303:errorcluster, error out=w311:errorcluster)
            n167 = local write "error out"(w303) -> ()
            n168 = call "Error Reported.vi"("Error"=w303) -> ()  [unwired: 10 in, 1 out]
            n169 = case shown="False" w304 {
              tunnel: [w318 _] -> w310
              tunnel: w306 -> [w316 _]
              tunnel: w303 -> [w317 _]
              frame False {
                n170 = disable-structure shown="Default" {
                  disable-tunnel: w317 -> [w319 _]
                  frame condition #0 (active) {
                    # "If the module is running standalone, then pop up an error dialog and call the \"Exit\" message."
                    n171 = call <vilib>:"Simple Error Handler.vi"("error in (no error)"=w319) -> ()  [unwired: 4 in, 5 out]
                  }
                  frame condition #1 {
                    # "To prevent the Simple Error Handler VI from being loaded (e.g. when deploying to a Real-Time target), add the Conditional Disable Symbol \"DQMH_Disable_SEH\" to your project and set it to TRUE."
                  }
                }
                n172 = call-poly <vilib>:"Delacor_lib_QMH_Enqueue Message (poly).vi"("Priority Message? (F)"=TRUE, "Message"="Exit", "Message Queue in"=w316) -> ("error out"=w318:errorcluster)  [unwired: 7 in, 1 out]
              }
              frame True {
                # "If the module was launched externally, calling the Error Reported broadcast VI is the only action performed by the \"Error\" message. The module's caller can then process the error appropriately."
              }
            }
            n173 = Merge Errors(w311, w310) -> (w309:errorcluster)
          }
          frame "Exit" {
            w324 = 91  # 91: not all Exit messages will have an argument
            w326 = TRUE  # Stop the VI
            # "send exit to controller"
            # "Release the message queue reference"
            # "#DQMH_CodeNeeded - Add any required cleanup code here."
            # "Exit - Exit the application."
            n174 = Variant To Data(error in=w334, type=T20 {"Origin"="", "Exit via Stop Module Req?"=FALSE, "Wait for Module to stop?"=FALSE} ("Stop Argument"), Variant=w325) -> (data=w322:T20, error out=w331:errorcluster)
            n175 = call <vilib>:"Clear Errors.vi"("error in (no error)"=w331, "specific error code to clear (0: all)"=w324) -> ("error out"=w333:errorcluster)  [unwired: 4 in, 1 out]
            n176 = control-ref of="This VI"() -> (w321:refnum<vi>)
            n177 = call-dynamic "Delacor_lib_QMH_Release Message Queue.vi"("error in"=w333, "Message Queue"=w328) -> ("error out"=w332:errorcluster)  [unwired: 9 in]
            n178 = call "Handle Exit.vi"("Stop Argument"=w322, "Admin in"=w320, "VI reference"=w321) -> ("error out"=w330:errorcluster)  [unwired: 7 in, 1 out]
            n179 = Merge Errors(w332, w330) -> (w329:errorcluster)
            n180 = call "Error Reported.vi"("Error"=w329) -> ()  [unwired: 10 in, 1 out]
            n181 = call "Stop Module.vi"() -> ()  [unwired: 11 in, 1 out]
          }
          frame Default {
            # "'Default' case only runs if there is a message that isn't defined in any of the other cases.  Output a programming error."
            n182 = call "Module Name--constant.vi"() -> ("Module Name"=w339:string)  [unwired: 11 in]
            n183 = Format Into String(format string="The invalid message string \"%s\" was received in the Message Handling Loop for module \"%s\".", w340, w339) -> (resulting string=w335:string)  [unwired: 2 in, 1 out]
            n184 = call <vilib>:"Error Cluster From Error Code.vi"("show call chain? (False)"=TRUE, "error message (\"\")"=w335, "error code (0)"=1) -> ("error out"=w342:errorcluster)  [unwired: 6 in]
            n185 = Merge Errors(w343, w342) -> (w344:errorcluster)
          }
        }
        n186 = call-dynamic "Delacor_lib_QMH_Error Handler - Message Handling Loop.vi"("error in"=w166, "Message Queue in"=w165) -> ("dup error in"=w167:errorcluster)  [unwired: 8 in, 1 out]
      }
    }
    frame Error {
      # "Synchronize Caller Events.vi will inform Start Module.vi that the module has launched and will let the code calling Start Module.vi register for broadcasts and would permit the caller receive the broadcast that an error occurred at launch time."
      n187 = call-dynamic "Delacor_lib_QMH_Release Message Queue.vi"("error in"=w352, "Message Queue"=w345) -> ("error out"=w351:errorcluster)  [unwired: 9 in]
      n188 = call "Synchronize Caller Events.vi"("Singleton Module Admin in"=w346) -> ("error out"=w353:errorcluster)  [unwired: 9 in, 1 out]
      n189 = call "Module Name--constant.vi"() -> ("Module Name"=w349:string)  [unwired: 11 in]
      n190 = Format Into String(format string="An error occurred during initialization. %s is no longer running.", w349) -> (resulting string=w347:string)  [unwired: 2 in, 1 out]
      n191 = Merge Errors(w351, w353) -> (w354:errorcluster)
      n192 = call "Error Reported.vi"("Additional Information"=w347, "Error"=w354) -> ()  [unwired: 9 in, 1 out]
    }
  }
  n193 = Merge Errors(w24, w27) -> (w23:errorcluster)
  n194 = call "Close Module.vi"("error in"=w23, "Module Admin in"=w19) -> ("error out"=w25:errorcluster, "External Launch"=w12:bool, "Module Admin out"=w13:refnum<class "Delacor_lib_QMH_Module Admin.lvclass">)  [unwired: 7 in]
  n195 = Unregister For Events(event registration refnum=w18, error in=w25) -> (error out=w22:errorcluster)
  "error out" <- w22
  n196 = case "External Launch?" shown="True" w12 {
    tunnel: w22 -> [_ w355]
    frame False {
    }
    frame True {
      n197 = case shown="No Error" w355 {
        frame No Error {
          n198 = invoke on="Invoke Node" class="VI" method="FP.Close"() -> ()  [unwired: 3 in, 3 out]
        }
        frame Error {
          n199 = disable-structure shown="Default" {
            frame condition #0 (active) {
              n200 = invoke class="VI" method="FP.Open"("Activate"=TRUE ("Activate?")) -> ()  [unwired: 4 in, 5 out]
            }
            frame condition #1 {
              # "Don't show panel on error if running inside a built EXE."
            }
          }
        }
      }
    }
  }
  n201 = local write "Module Admin"(w13) -> ()
